vi "initilizeEMCY.vi"(8 "error in (no error)":errorcluster, 10 "interface object in":refnum<k20>, 11 "MotorControllerClass in":refnum<class "MotorControllerClass.lvclass">) -> (0 "error out":errorcluster, 1 "emergency object out":refnum<k20>, 2 "interface object out":refnum<k20>, 3 "MotorControllerClass out":refnum<class "MotorControllerClass.lvclass">)   [LabVIEW 2018, in "MotorControllerClass.lvclass"]
uses:
  MotorControllerClass.lvclass
  <vilib>/CANopenLib/CANOPEN.llb/CANopen Emergency Create.vi
  <vilib>/CANopenLib/CANOPEN.llb/CANopen Emergency Start.vi
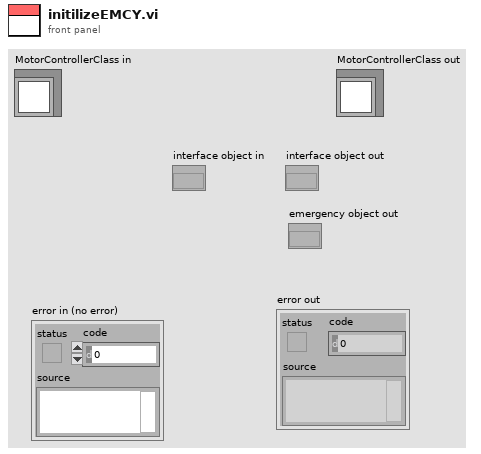
[diagram p1: front panel]
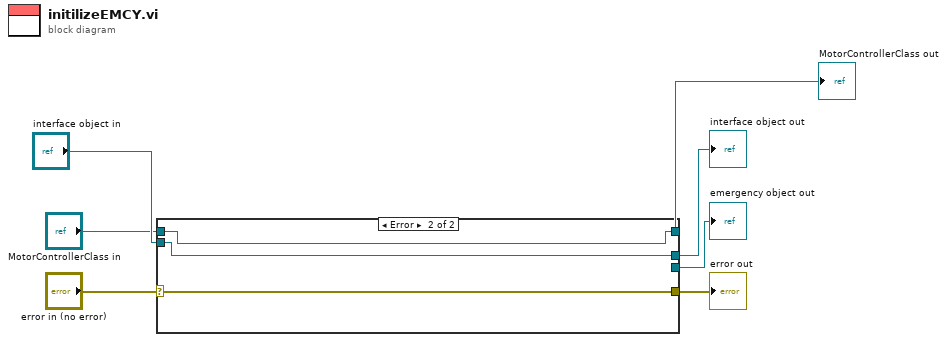
[diagram p0: block diagram]
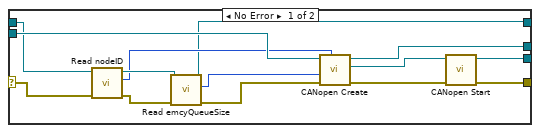
[diagram p2: hidden frame]
diagram:
  n1 = case shown="Error" "error in (no error)" {
    selector: "error in (no error)" -> [w15 w24]
    tunnel: [w17 w24] -> w6
    tunnel: "MotorControllerClass in" -> [w9 w22]
    tunnel: "interface object in" -> [w19 w23]
    tunnel: [w18 w23] -> w4
    tunnel: [w16 _] -> w3
    tunnel: [w8 w22] -> w1
    frame No Error {
      n2 = call-dynamic "Read nodeID.vi"("error in (no error)"=w15, "MotorControllerClass in"=w9) -> ("error out"=w13:errorcluster, "nodeID"=w12:u8, "MotorControllerClass out"=w14:refnum<class "MotorControllerClass.lvclass">)  [unwired: 7 in]
      n3 = call-dynamic "Read emcyQueueSize.vi"("error in (no error)"=w13, "MotorControllerClass in"=w14) -> ("error out"=w10:errorcluster, "emcyQueueSize"=w11:u16, "MotorControllerClass out"=w8:refnum<class "MotorControllerClass.lvclass">)  [unwired: 7 in]
      n4 = call-poly <vilib>:"CANopen Create.vi"("node-ID"=w12, "error in (no error)"=w10, "buffer size (0)"=w11, "interface object in"=w19) -> ("error out"=w20:errorcluster, "emergency object out"=w21:refnum<k20>, "interface object out"=w18:refnum<k20>)  [unwired: 5 in]
      n5 = call-poly <vilib>:"CANopen Start.vi"("error in (no error)"=w20, "emergency object in"=w21) -> ("error out"=w17:errorcluster, "emergency object out"=w16:refnum<k20>)  [unwired: 8 in]
    }
    frame Error {
    }
  }
  "error out" <- w6
  "interface object out" <- w4
  "emergency object out" <- w3
  "MotorControllerClass out" <- w1
